vi "Encode Parameters into Words for Labels in a Channel.vi"(7 "reset index":bool, 8 "error in (no error)":errorcluster, 9 "labels settings for RT in":T1[](array[typedef]) {"Label Timestamp Channel Data Reference" format="%.0x"; "Word Initial Raw Value" format="%032.0f"; "Label Disable/Trigger Channel Reference" format="%.0x"; "parameter driver data"."Tx parameter refs" format="%.0x"; "SDI" format="%02b"; "label" format="%.0o"}, 11 "Parameter Values in":dbl[](array[numeric])) -> (0 "error out":errorcluster, 1 "labels settings for RT out":T1[](array[typedef]) {"Label Timestamp Channel Data Reference" format="%.0x"; "Word Initial Raw Value" format="%032.0f"; "Label Disable/Trigger Channel Reference" format="%.0x"; "parameter driver data"."Tx parameter refs" format="%.0x"; "SDI" format="%02b"; "label" format="%.0o"}, 2 "data words out":u32[](array[numeric]))   [LabVIEW 2020, in "AIM ARINC 429 Engine.lvlib" / "Implementation.lvlib" / "Tx Scheduled Labels Execution Unit.lvclass"]
uses:
  Tx Scheduled Labels Execution Unit.lvclass
  Shared/RT Label Settings.ctl
  Shared/Label.ctl
  Shared/RT Parameters.ctl
  Shared/Parameter Definition.ctl
  <vilib>/NI/NI VeriStand Encoding and Decoding/Encoding.ctl
  <vilib>/NI VeriStand/Custom Device API/Custom Device Item Ref.ctl
  Shared/Transfer Type.ctl
  <vilib>/NI VeriStand/Custom Device API/Data Reference.ctl
  Shared/Encode Parameter and Update Word (32-bit).vi/1445f95d-237d-4fc6-96b9-8992d347f513.vi
  Shared/Encode Parameter and Update Word (32-bit).vi/6b8853f0-8e5d-49e3-9391-4d3f8e5314b0.vi
  Shared/Encode Parameter and Update Word (32-bit).vi/2babc4f4-546e-4d35-846d-a4a1fbac0249.vi
  Shared/Encode Parameter and Update Word (32-bit).vi/1445f95d-237d-4fc6-96b9-8992d347f513.vi/9377bb8f-44b5-4a8f-87f1-966fd5a9edcc.vi
  Shared/Encode Parameter and Update Word (32-bit).vi/1445f95d-237d-4fc6-96b9-8992d347f513.vi/e95d9d1f-307c-44d6-9f26-c3f519a4990d.vi
  Shared/Encode Parameter and Update Word (32-bit).vi/1445f95d-237d-4fc6-96b9-8992d347f513.vi/0c23f515-4369-4514-bc3d-4444e6b437b2.vi
  Shared/Encode Parameter and Update Word (32-bit).vi/6b8853f0-8e5d-49e3-9391-4d3f8e5314b0.vi/136dcdcb-2dd3-4a4d-a796-a8f7a3f8e1ac.vi
  Shared/Encode Parameter and Update Word (32-bit).vi/6b8853f0-8e5d-49e3-9391-4d3f8e5314b0.vi/a54b505c-1216-4ef4-8378-3ceda9d188df.vi
  <vilib>/NI/NI VeriStand Encoding and Decoding/Get Bits Per Digit from Base.vi
  <vilib>/NI/NI VeriStand Encoding and Decoding/Encoding and Decoding.lvlib
  <vilib>/NI VeriStand/Custom Device API/Custom Device API.lvlib
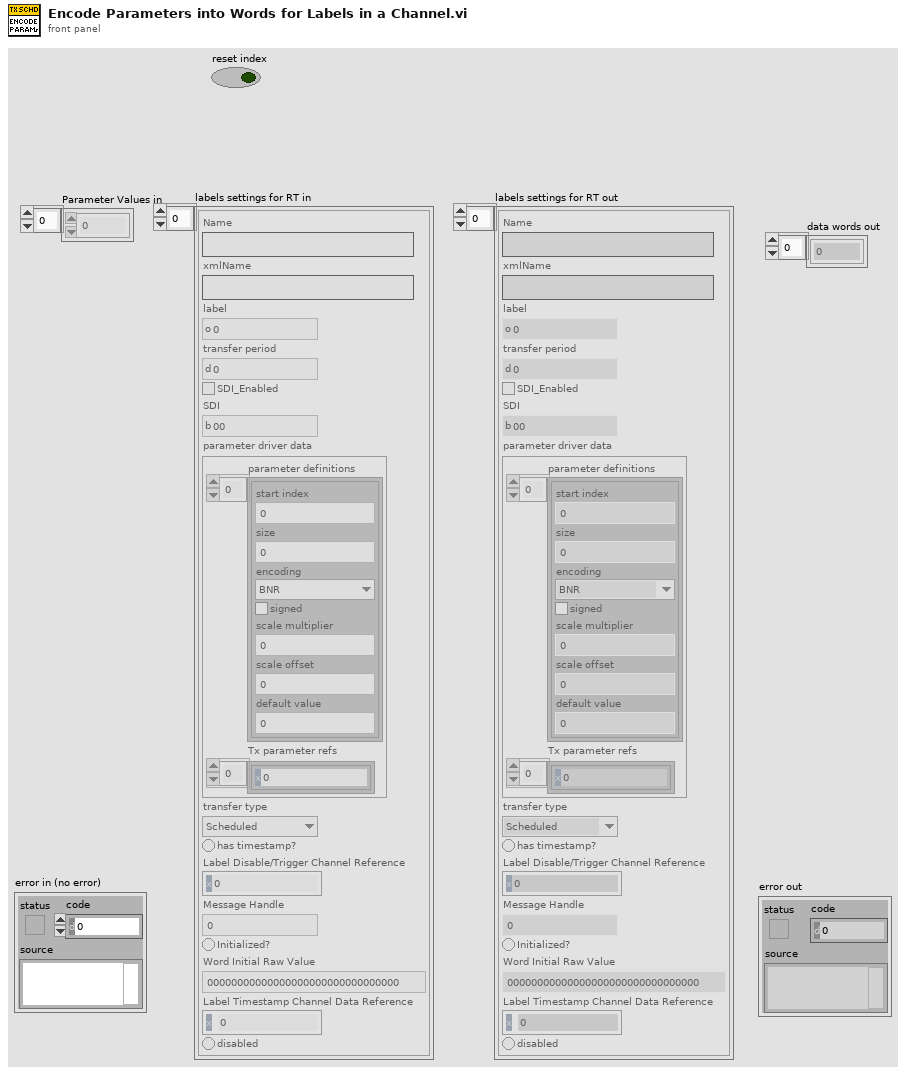
[diagram p1: front panel]
types:
  T1 = typedef "RT Label Settings.ctl" = cluster{"Name":string, "xmlName":string, "label":T2, "transfer period":u32, "SDI_Enabled":bool, "SDI":u8, "parameter driver data":T3, "transfer type":T7, "has timestamp?":bool, "Label Disable/Trigger Channel Reference":T6, "Message Handle":u64, "Initialized?":bool, "Word Initial Raw Value":u32, "Label Timestamp Channel Data Reference":T8, "disabled":bool}
  T2 = typedef "Label.ctl" = u8
  T3 = typedef "RT Parameters.ctl" = cluster{"parameter definitions":T4[], "Tx parameter refs":T6[]}
  T4 = typedef "Parameter Definition.ctl" = cluster{"start index":i32, "size":i32, "encoding":T5, "signed":bool, "scale multiplier":dbl, "scale offset":dbl, "default value":dbl}
  T5 = typedef "Encoding and Decoding.lvlib/Encoding.ctl" = enum16{"BNR", "BCD", "Discrete"}
  T6 = typedef "Custom Device API.lvlib/Custom Device Item Ref.ctl" = u64
  T7 = typedef "Transfer Type.ctl" = enum16{"Scheduled", "Acyclic", "Block", "Strobe"}
  T8 = typedef "Custom Device API.lvlib/Data Reference.ctl" = i32
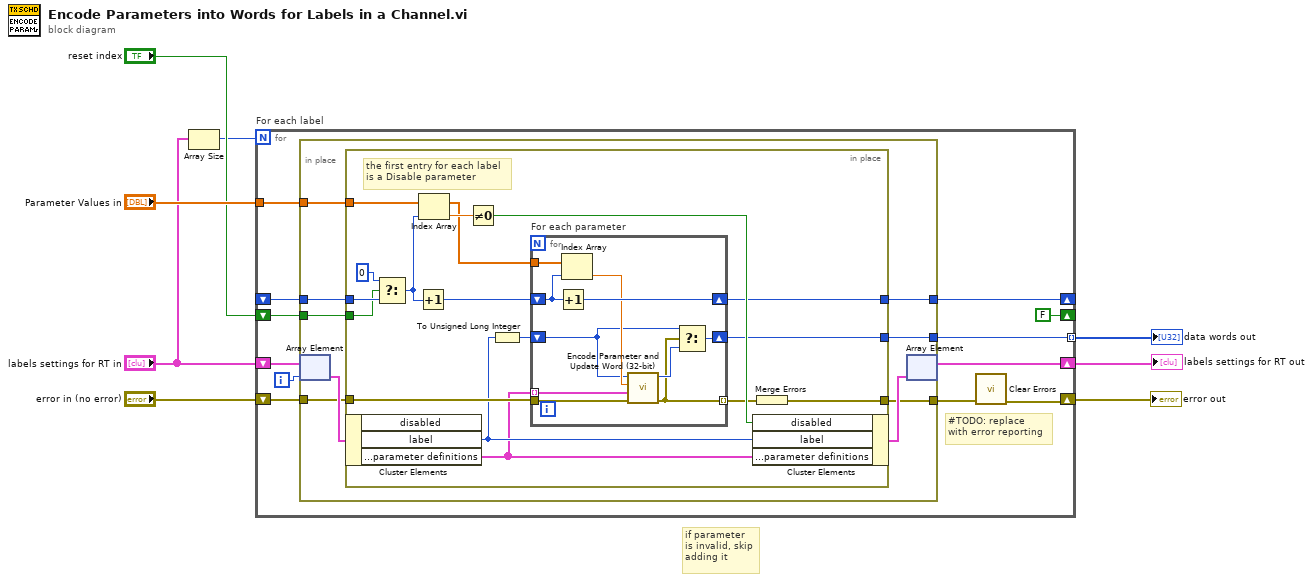
[diagram p0: block diagram]
diagram:
  # "if parameter\nis invalid, skip\nadding it"
  n1 = Array Size(array="labels settings for RT in") -> (size(s)=w2:i32)
  n2 = for "For each label" {
    N: w2 -> [_]
    shift-right: [w9] -> w8
    shift-left: "error in (no error)" -> [w16]
    shift-right: [FALSE ("reset index")] -> _
    shift-left: "reset index" -> [w14]
    tunnel: "Parameter Values in" -> [w18]
    shift-right: [w15] -> _
    shift-left: _ -> [w17]
    tunnel: [w12] -> w4 mode=indexing
    shift-right: [w11] -> w3
    shift-left: "labels settings for RT in" -> [w20]
    i -> [w19]
    # "#TODO: replace\nwith error reporting"
    n3 = in-place {
      in-place-border: w18 -> [w27]
      in-place-border: w17 -> [w26]
      in-place-border: w16 -> [w25]
      in-place-border: [w24] -> w15
      in-place-border: w14 -> [w23]
      in-place-border: [w22] -> w12
      in-place-border: [w21] -> w10
      n4 = in-place-array #1(w20, w19) -> (w29:T1)
      n5 = in-place {
        in-place-border: w27 -> [w40]
        in-place-border: w26 -> [w44]
        in-place-border: w25 -> [w39]
        in-place-border: [w36] -> w24
        in-place-border: w23 -> [w35]
        in-place-border: [w34] -> w22
        in-place-border: [w30] -> w21
        # "the first entry for each label\nis a Disable parameter"
        n6 = in-place-cluster #2(w29) -> ("label"=w33:T2, "parameter driver data.parameter definitions"=w32:T4[])  [unwired: 1 out]
        n7 = Select(t=0 ("index"), s=w35, f=w44) -> (s? t:f=w43:i32)
        n8 = Increment(x=w43) -> (x+1=w41:i32)
        n9 = Index Array(array=w40, index=w43) -> (element=w42:dbl)
        n10 = Not Equal To 0?(x=w42) -> (x != 0?=w38:bool)
        n11 = To Unsigned Long Integer(number=w33) -> (unsigned 32bit integer=w37:u32)
        n12 = for "For each parameter" {
          shift-right: [w53] -> w36
          shift-left: w41 -> [w54]
          tunnel: w40 -> [w55]
          tunnel: w32 -> [w51] mode=indexing
          shift-right: [w47] -> w34
          shift-left: w37 -> [w48]
          tunnel: w39 -> [w50]
          tunnel: [w46] -> w31 mode=indexing
          n13 = Increment(x=w54) -> (x+1=w53:i32)
          n14 = Index Array(array=w55, index=w54) -> (element=w52:dbl)
          n15 = call "Encode Parameter and Update Word (32-bit).vi"("error in"=w50, "parameter definition"=w51, "parameter value"=w52, "word in"=w48) -> ("error out"=w46:errorcluster, "word out"=w49:u32)  [unwired: 6 in]
          n16 = Select(t=w48, s=w46, f=w49) -> (s? t:f=w47:u32)
        }
        n17 = in-place-cluster #2("disabled"=w38, "label"=w33, "parameter driver data.parameter definitions"=w32) -> (w28:T1)
        n18 = Merge Errors(w31) -> (w30:errorcluster)
      }
      n19 = in-place-array #1(w28) -> (w11:T1[])  [unwired: 1 out]
    }
    n20 = call <vilib>:"Clear Errors.vi"("error in (no error)"=w10) -> ("error out"=w9:errorcluster)  [unwired: 5 in, 1 out]
  }
  "data words out" <- w4
  "error out" <- w8
  "labels settings for RT out" <- w3
